vi "Evaluate Part 2.vi"() -> ()   [LabVIEW 2021]
uses:
  Proto/Proto.lvclass
panel:
  out "x*y":u64
  out "size(s) 2":i32
  out "Intensity Graph":i32[][](graph)
  in  "Steps":i32
  in  "Input":string
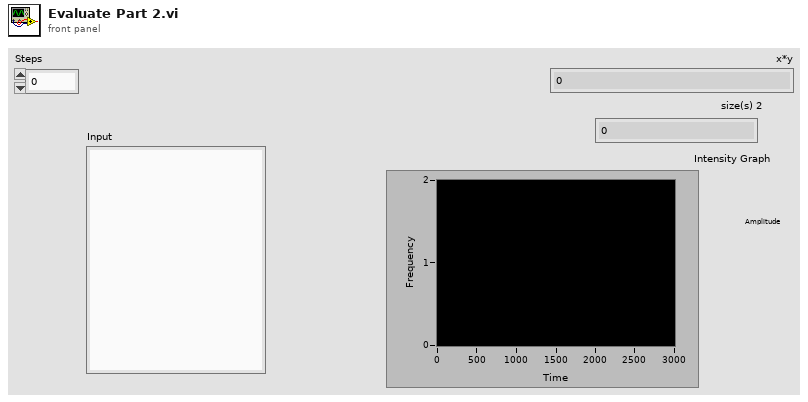
[diagram p1: front panel]
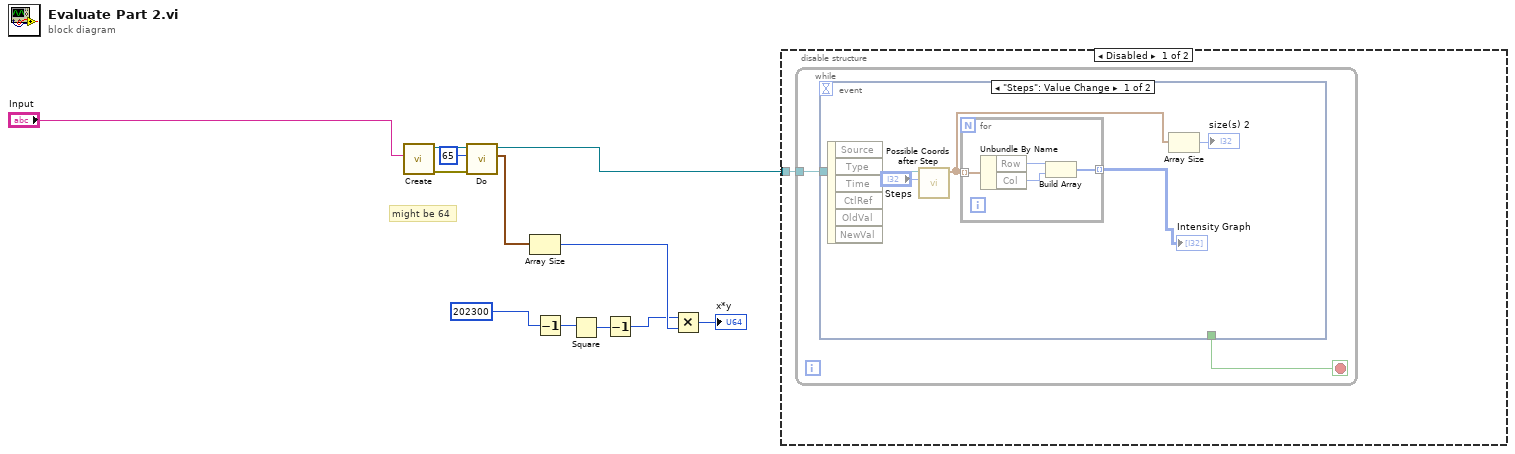
[diagram p0: block diagram]
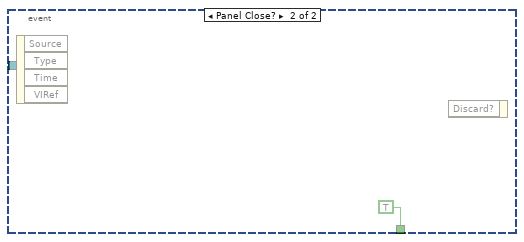
[diagram p2: hidden frame]
diagram:
  # "might be 64"
  n1 = call "Create.vi"("Input"="Input") -> ("error out"=w11:errorcluster, "Proto"=w12:refnum<class "Proto.lvclass">)  [unwired: 9 in]
  n2 = call "Do.vi"("error in (no error)"=w11, "Steps"=65, "Proto In"=w12) -> ("Possible Coords"=w7:cluster{"Row":i32, "Col":i32}[], "Proto Out"=w8:refnum<class "Proto.lvclass">)  [unwired: 6 in, 1 out]
  n3 = Array Size(array=w7) -> (size(s)=w3:i32)
  n4 = Decrement(x=u64 202300 ("y")) -> (x-1=w6:u64)
  n5 = Square(x=w6) -> (x^2=w5:u64)
  n6 = Decrement(x=w5) -> (x-1=w1:u64)
  n7 = Multiply(x=w1, y=w3) -> (x*y=→"x*y":u64)
  n8 = disable-structure shown="Disabled" {
    disable-tunnel: w8 -> [w13 _]
    frame Disabled {
      n9 = while {
        tunnel: w13 -> [w15]
        stop <- w14 stop-if-true
        n10 = event shown="[0] \"Steps\": Value Change" {
          selector: _ -> [_ _]
          dyn-events: _ -> [_ _]
          timeout: _ -> [_ _]
          tunnel: w15 -> [w20 _]
          tunnel: [_ TRUE] -> w14
          event "Steps": Value Change {
            n11 = event-data() -> ()  [unwired: 1 in, 6 out]
            n12 = call "Possible Coords after Step.vi"("Steps"="Steps", "Proto in"=w20) -> ("Array"=w16:cluster{"Row":i32, "Col":i32}[])  [unwired: 9 in]
            n13 = for {
              tunnel: w16 -> [w24] mode=indexing
              tunnel: [w21] -> w18 mode=indexing
              n14 = Unbundle By Name(w24) -> ("Row"=w23:i32, "Col"=w22:i32)
              n15 = Build Array(w23, w22) -> (w21:i32[])
            }
            "Intensity Graph" <- w18
            n16 = Array Size(array=w16) -> (size(s)=→"size(s) 2":i32)
          }
          event Panel Close? {
            n17 = event-data() -> ()  [unwired: 1 in, 4 out]
            n18 = event-data() -> ()  [unwired: 2 in, 1 out]
          }
        }
      }
    }
    frame Enabled {
    }
  }
